vi "pb_close.vi"(8 "error in (no error)":errorcluster, 11 "path in":path=path "C:/Program Files/SpinCore/SpinAPI/dll/spinapi.dll") -> (0 "error out":errorcluster, 3 "path out":path)   [LabVIEW 2013, in "SpinAPI-20140801.lvlib"]
uses:
  SpinAPI-20140801.lvlib
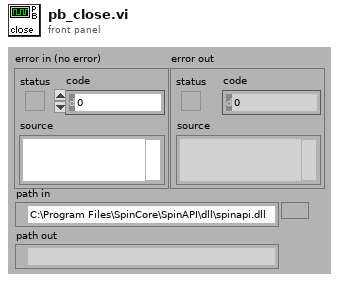
[diagram p1: front panel]
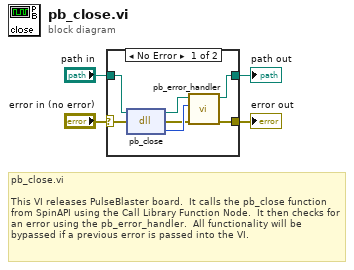
[diagram p0: block diagram]
diagram:
  # "pb_close.vi\n\nThis VI releases PulseBlaster board.  It calls the pb_close function from SpinAPI using the Call Library Function Node.  It then checks for an error using the pb_error_handler.  All functionality will be bypassed if a previous error is passed into the VI."
  n1 = case shown="No Error" "error in (no error)" {
    selector: "error in (no error)" -> [w11 w13]
    tunnel: [w7 w13] -> w3
    tunnel: "path in" -> [w6 w12]
    tunnel: [w5 w12] -> w1
    frame No Error {
      n2 = dll-call lib="C:/Program Files/SpinCore/SpinAPI/dll/spinapi.dll" fn="pb_close"(path in=w6, error in=w11) -> (path out=w9:path, error out=w8:errorcluster, "return type"=w10:i32)  [unwired: 1 in]
      n3 = call "pb_error_handler.vi"("error in (no error)"=w8, "return code"=w10, "path in"=w9) -> ("error out"=w7:errorcluster, "path out"=w5:path)  [unwired: 7 out]
    }
    frame Error {
    }
  }
  "error out" <- w3
  "path out" <- w1
